vi "Host-Top-Level.vi"() -> ()   [LabVIEW 2017]
uses:
  State.ctl
  <vilib>/FPGAPlugInAG/PXIe-6592R/niLvFpga_Open_PXIe-6592R.vi
  <vilib>/rvi/interface/common/dynamic/niFpgaDynamicAddResources.vi
  <vilib>/Utility/error.llb/Error Cluster From Error Code.vi
  <vilib>/rvi/errors/niLvFpgaAdjustHostInterfaceError.vi
  <vilib>/FPGAPlugInAG/Dynamic/niLvFpga_Close_Dynamic.vi
  <vilib>/rvi/interface/nirviOpenFPGA/nirviOpenFPGA.xnode
  FPGA Bitfiles/04lwIpExercisor_FPGATarget_Fpga-Exercisor-T_vFkl61iGjK8.lvbitx
  PXIe-6592/Fpga-Exercisor-Top.vi
  <vilib>/rvi/interface/nirviMethod/nirviMethod.xnode
  <vilib>/rvi/interface/nirviReadWriteControl/nirviReadWriteControl.xnode
  <vilib>/rvi/interface/nirviCloseFPGA/nirviCloseFPGA.xnode
  <vilib>/rvi/errors/niLvFpgaMergeErrorWithErrorCode.vi
  <vilib>/FPGAPlugInAG/Dynamic/niLvFpga_ReadFifo_Dynamic.vi
  <vilib>/rvi/interface/Simulation/niFpgaSimulationCallBeginRW.vi
  <vilib>/FPGAPlugInAG/Dynamic/niLvFpga_WriteFifo_Dynamic.vi
  NiFpgaLv.dll
panel:
  in  "Read FIFO #2":bool
  in  "Read FIFO #1":bool
  in  "Interrupt #1":bool
  in  "Interrupt #0":bool
  out "AXI_STR_RXD_tready 2":bool
  out "tvalid 2":bool
  out "tdata 2":u32
  out "tlast 2":bool
  out "AXI_STR_RXD_tready_Count 2":u16
  out "tvalid_Count 2":u16
  out "tlast_Count 2":u16
  out "tdata_LastNonZero 2":u32
  out "Read Data 2":u32[](array[numeric]) format="%.0x"
  in  "DataToSend 2":u32[](array[numeric])=[240, 241, 242, 243, 244, 245] format="%.0x"
  in  "Send to FIFO #2":bool
  out "GPO2 Channel 2":u32
  in  "GPO2 Channel 1":u32
  in  "GPIO Write-Read #2":bool
  out "GPO1 Channel 1":u32 format="%.0x"
  out "error out":errorcluster
  out "GPO2 Channel 2":u32 format="%.0x"
  in  "Read all GPO":bool
  out "GPO1 Channel 2":u32
  in  "GPO1 Channel 1":u32
  in  "GPIO Write-Read #1":bool
  out "Read Data":u32[](array[numeric]) format="%.0x"
  in  "DataToSend":u32[](array[numeric])=[240, 241, 242, 243, 244, 245] format="%.0x"
  in  "Send to FIFO #1":bool
  in  "Stop":bool
  in  "error in":errorcluster
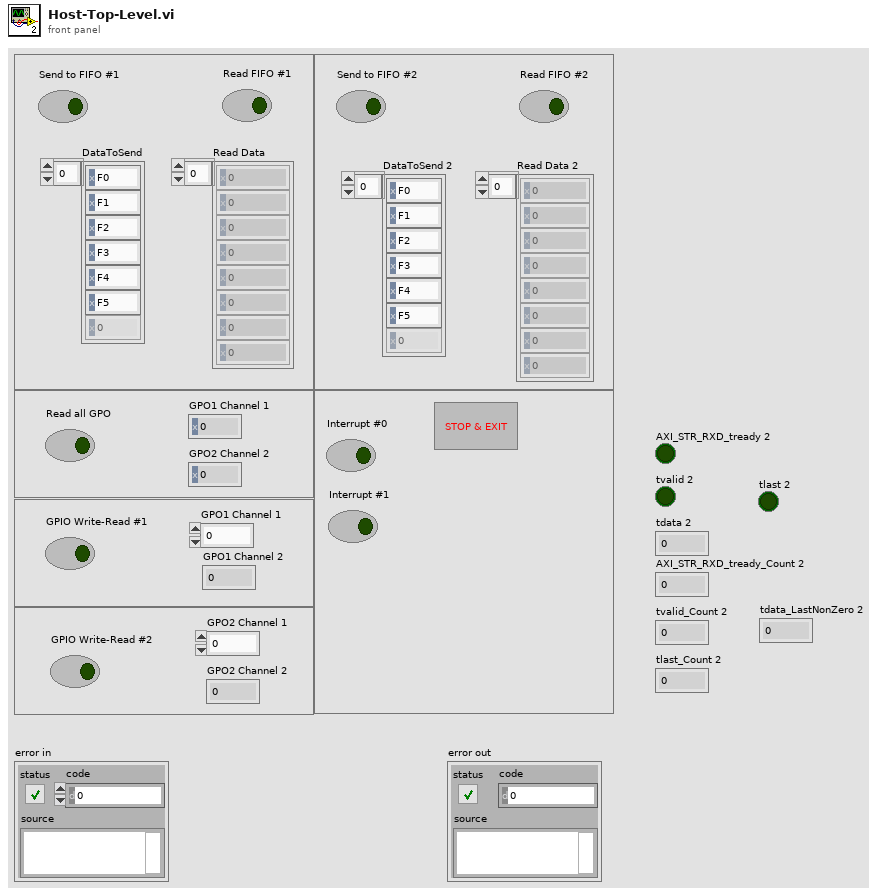
[diagram p1: front panel]
types:
  T1 = typedef "State.ctl" = enum16{"Initialize", "Idle", "Read #1", "Read #2", "Read Status", "Exit"}
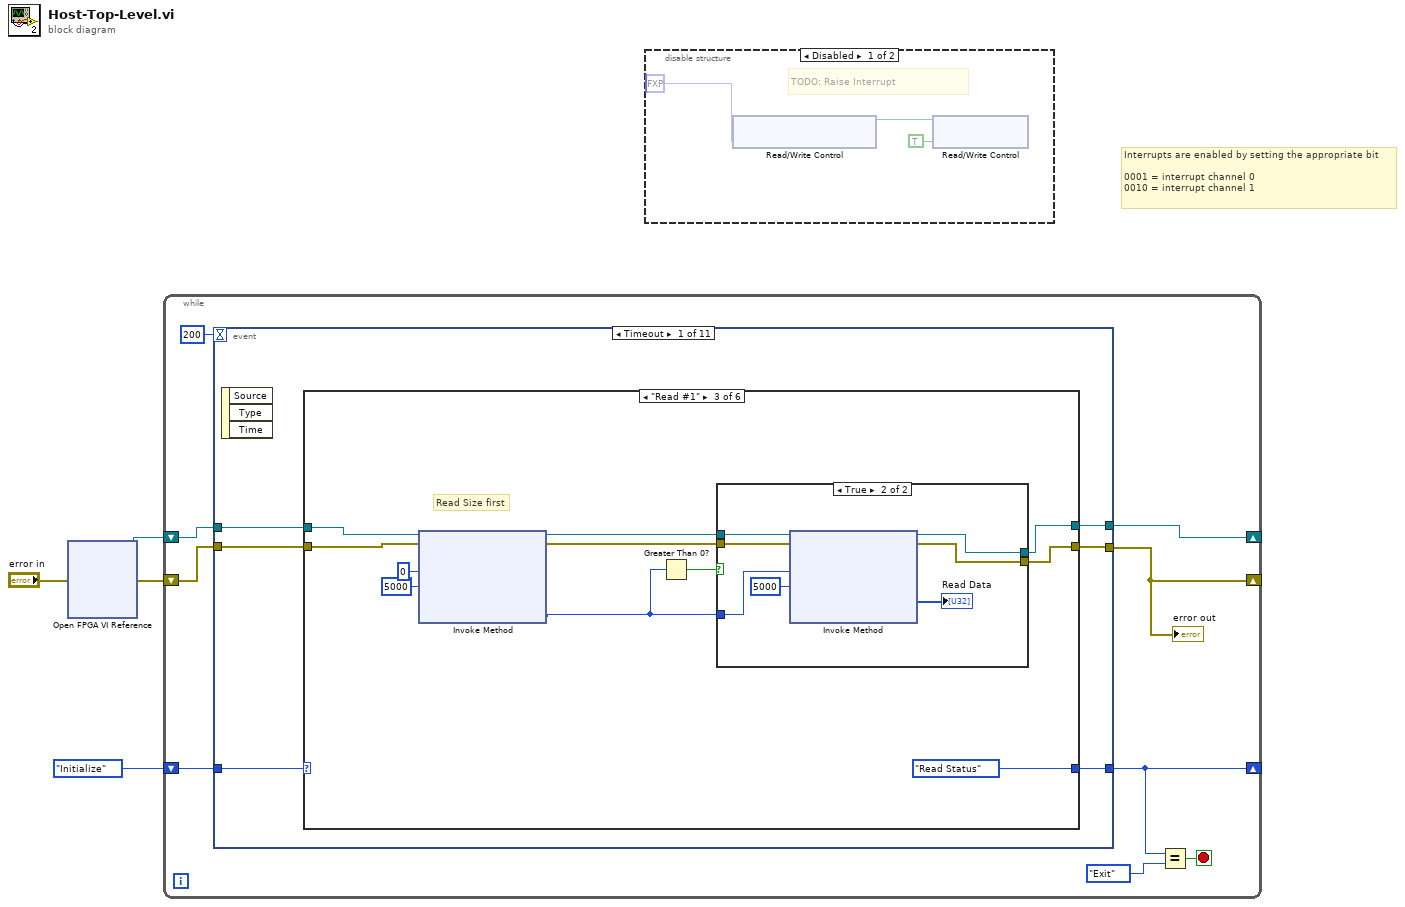
[diagram p0: block diagram]
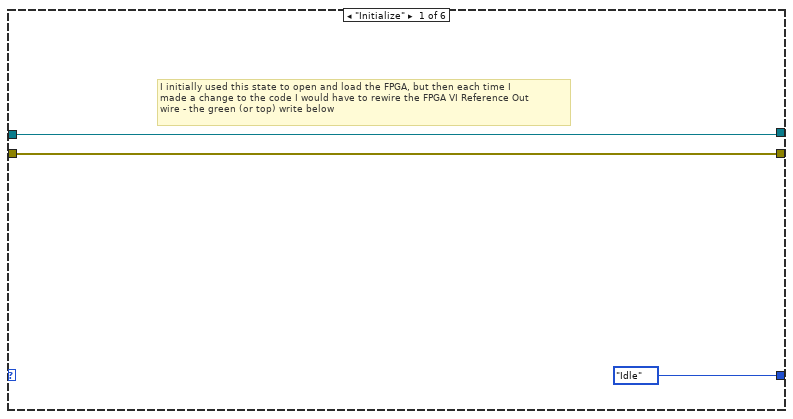
[diagram p3: hidden frame]
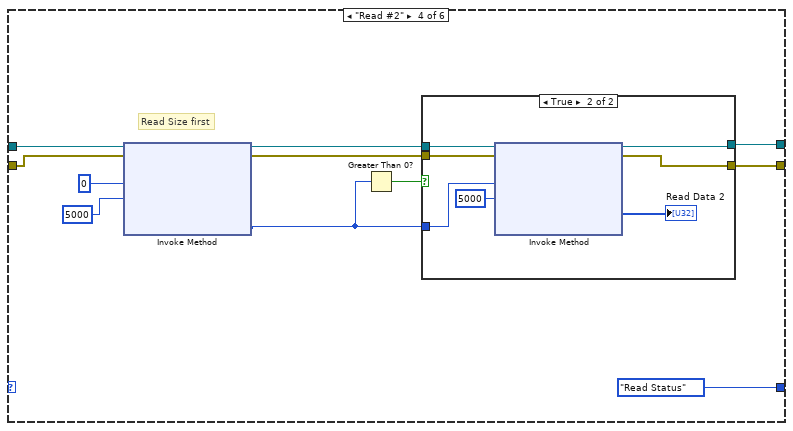
[diagram p6: hidden frame]
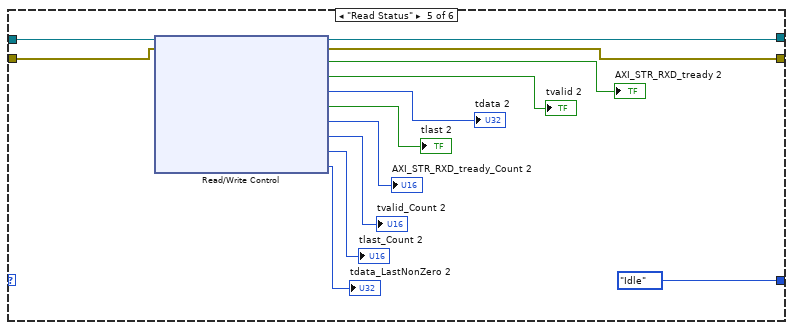
[diagram p8: hidden frame]
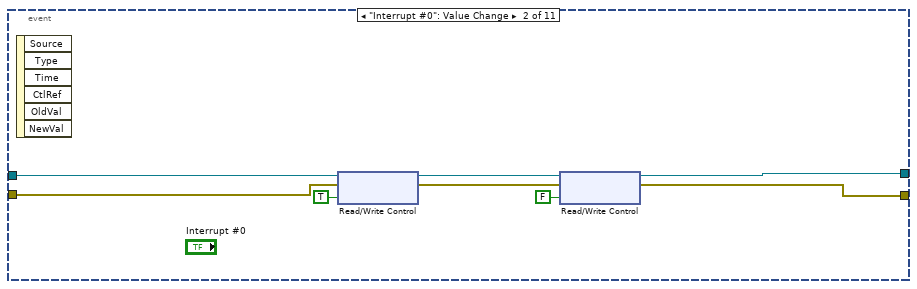
[diagram p10: hidden frame]
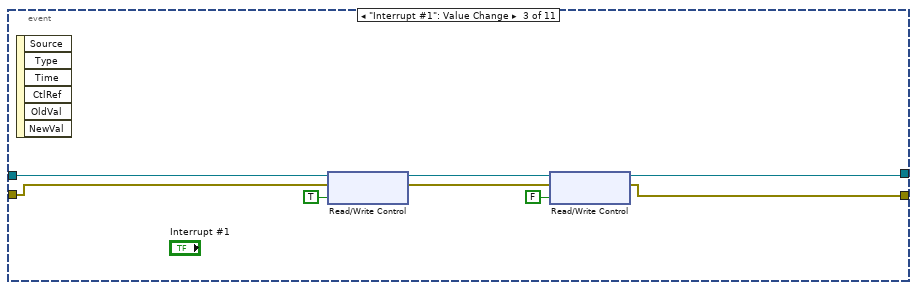
[diagram p11: hidden frame]
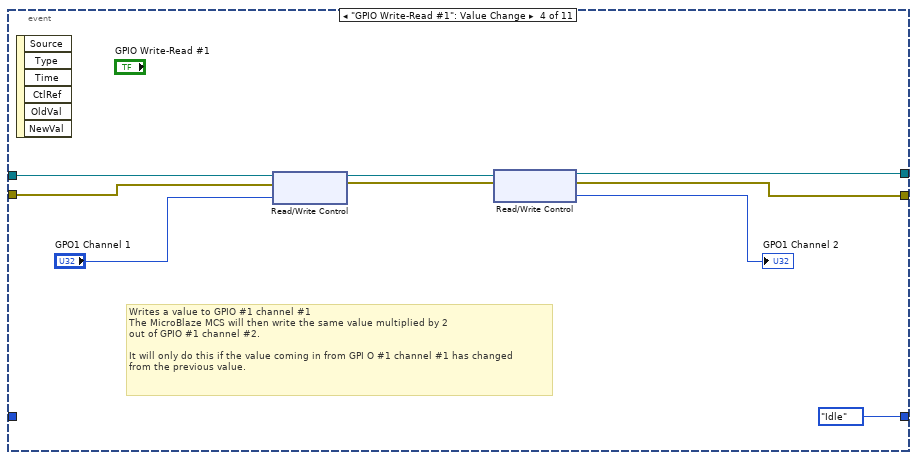
[diagram p12: hidden frame]
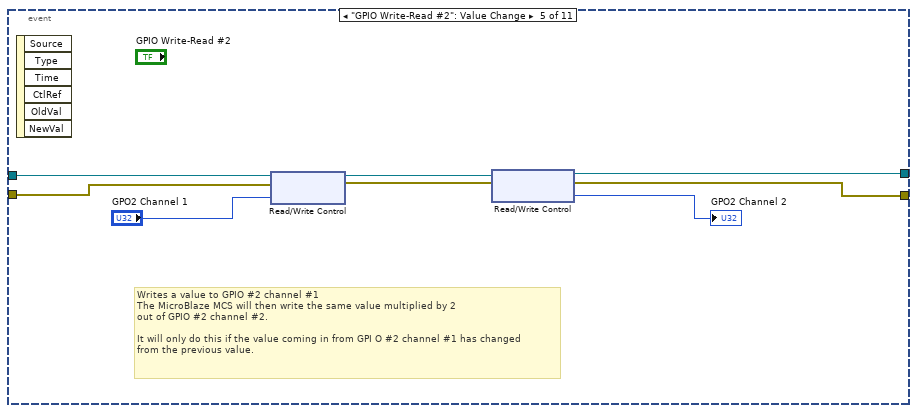
[diagram p13: hidden frame]
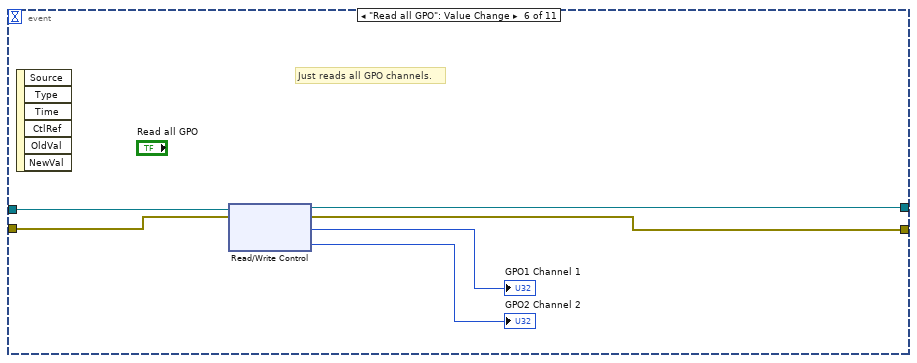
[diagram p14: hidden frame]
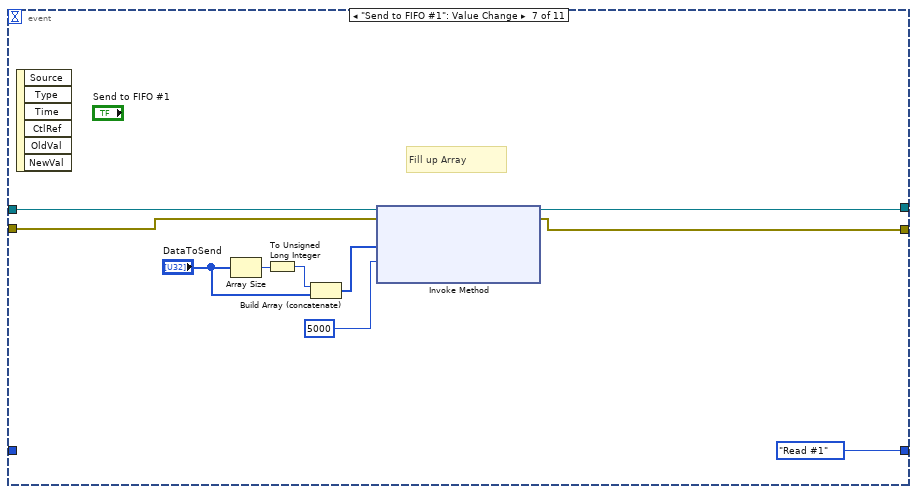
[diagram p15: hidden frame]
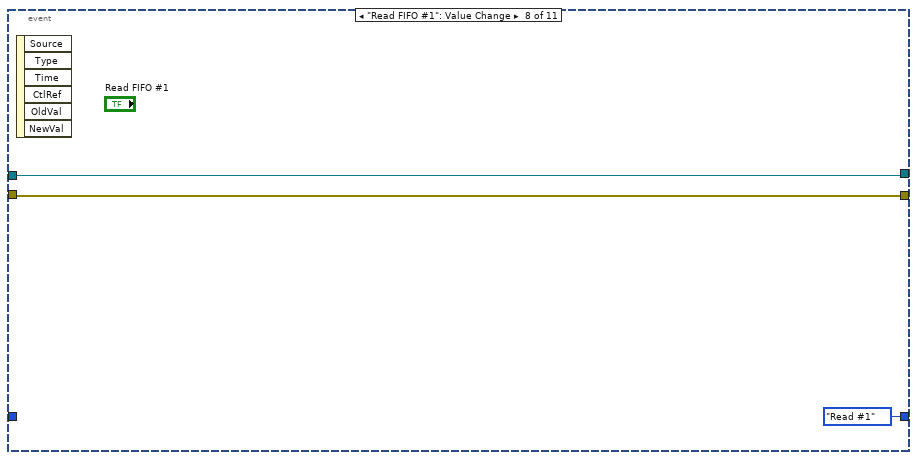
[diagram p16: hidden frame]
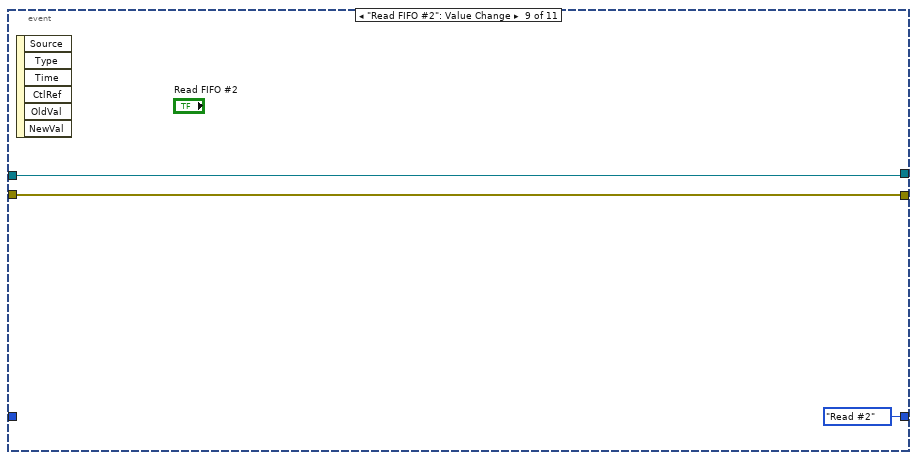
[diagram p17: hidden frame]
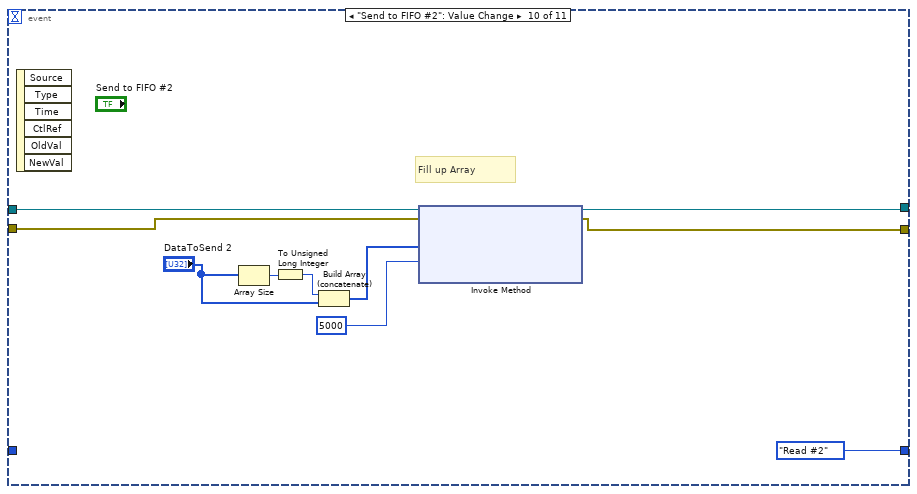
[diagram p18: hidden frame]
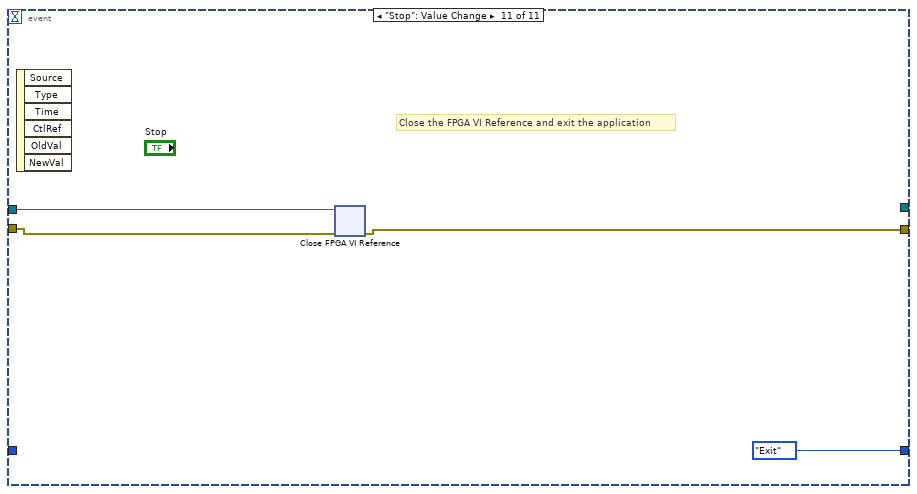
[diagram p19: hidden frame]
diagram:
  # "Interrupts are enabled by setting the appropriate bit\n\n0001 = interrupt channel 0\n0010 = interrupt channel 1"
  n1 = xnode "Open FPGA VI Reference"("error in"="error in") -> ("FPGA VI Reference Out"=w4:refnum<k20>, "error out"=w2:errorcluster)  [unwired: 1 in]
  n2 = while {
    shift-right: [w7] -> _
    shift-left: State."Initialize" ("Enum") -> [w13]
    shift-right: [w8] -> _
    shift-left: w2 -> [w9]
    shift-right: [w6] -> _
    shift-left: w4 -> [w5]
    stop <- w11 stop-if-true
    n3 = event shown="[0] Timeout" {
      selector: _ -> [_ _ _ _ _ _ _ _ _ _ _]
      dyn-events: _ -> [_ _ _ _ _ _ _ _ _ _ _]
      timeout: 200 -> [_ _ _ _ _ _ _ _ _ _ _]
      tunnel: [w17 _ _ State."Idle" ("Enum") _ _ State."Read #1" ("Enum") State."Read #1" ("Enum") State."Read #2" ("Enum") State."Read #2" ("Enum") State."Exit" ("Enum")] -> w7
      tunnel: w13 -> [w16 _ _ _ _ _ _ _ _ _ _]
      tunnel: w5 -> [w15 w89 w93 w105 w112 w120 w130 w132 w134 w146 w150]
      tunnel: w9 -> [w19 w83 w92 w104 w111 w119 w129 w131 w135 w145 w149]
      tunnel: [w18 w84 w91 w100 w110 w118 w122 w131 w135 w138 w148] -> w8
      tunnel: [w14 w85 w90 w98 w107 w117 w121 w132 w134 w139 _] -> w6
      event Timeout {
        n4 = event-data() -> ()  [unwired: 1 in, 3 out]
        n5 = case shown="\"Read #1\"" w16 {
          selector: w16 -> [_ w24 _ _ _ w80]
          tunnel: w19 -> [w21 w25 w36 w56 w68 w81]
          tunnel: [w21 w25 w31 w51 w67 w81] -> w18
          tunnel: w15 -> [w20 w23 w27 w47 w77 w79]
          tunnel: [State."Idle" ("Enum") w24 State."Read Status" ("Enum") State."Read Status" ("Enum") State."Idle" ("Enum") w80] -> w17
          tunnel: [w20 w23 w28 w48 w66 w79] -> w14
          frame "Initialize" {
            # "I initially used this state to open and load the FPGA, but then each time I \nmade a change to the code I would have to rewire the FPGA VI Reference Out \nwire - the green (or top) write below"
          }
          frame "Idle", Default {
          }
          frame "Read #1" {
            # "Read Size first"
            n6 = xnode "Invoke Method"("FPGA VI Reference In"=w27, "error in"=w36, "Number of Elements"=u32 0, "Timeout (ms)"=5000) -> ("FPGA VI Reference Out"=w32:refnum<k20>, "error out"=w33:errorcluster, "Elements Remaining"=w26:u32)  [unwired: 1 out]
            n7 = Greater Than 0?(x=w26) -> (x > 0?=w29:bool)
            n8 = case shown="True" w29 {
              tunnel: w33 -> [w38 w45]
              tunnel: w32 -> [w37 w44]
              tunnel: [w38 w42] -> w31
              tunnel: [w37 w41] -> w28
              tunnel: w26 -> [_ w39]
              frame False {
              }
              frame True {
                n9 = xnode "Invoke Method"("FPGA VI Reference In"=w44, "error in"=w45, "Number of Elements"=w39, "Timeout (ms)"=5000) -> ("FPGA VI Reference Out"=w41:refnum<k20>, "error out"=w42:errorcluster, "Data"=→"Read Data":u32[])  [unwired: 1 out]
              }
            }
          }
          frame "Read #2" {
            # "Read Size first"
            n10 = xnode "Invoke Method"("FPGA VI Reference In"=w47, "error in"=w56, "Number of Elements"=u32 0, "Timeout (ms)"=5000) -> ("FPGA VI Reference Out"=w52:refnum<k20>, "error out"=w53:errorcluster, "Elements Remaining"=w46:u32)  [unwired: 1 out]
            n11 = Greater Than 0?(x=w46) -> (x > 0?=w49:bool)
            n12 = case shown="True" w49 {
              tunnel: w53 -> [w58 w65]
              tunnel: w52 -> [w57 w64]
              tunnel: [w58 w62] -> w51
              tunnel: [w57 w61] -> w48
              tunnel: w46 -> [_ w60]
              frame False {
              }
              frame True {
                n13 = xnode "Invoke Method"("FPGA VI Reference In"=w64, "error in"=w65, "Number of Elements"=w60, "Timeout (ms)"=5000) -> ("FPGA VI Reference Out"=w61:refnum<k20>, "error out"=w62:errorcluster, "Data"=→"Read Data 2":u32[])  [unwired: 1 out]
              }
            }
          }
          frame "Read Status" {
            n14 = xnode "Read/Write Control"("FPGA VI Reference In"=w77, "error in"=w68) -> ("FPGA VI Reference Out"=w66:refnum<k20>, "error out"=w67:errorcluster, "AXI_STR_RXD_tready 2"=→"AXI_STR_RXD_tready 2":bool, "tvalid 2"=→"tvalid 2":bool, "tdata 2"=→"tdata 2":u32, "tlast 2"=→"tlast 2":bool, "AXI_STR_RXD_tready_Count 2"=→"AXI_STR_RXD_tready_Count 2":u16, "tvalid_Count 2"=→"tvalid_Count 2":u16, "tlast_Count 2"=→"tlast_Count 2":u16, "tdata_LastNonZero 2"=→"tdata_LastNonZero 2":u32)
          }
          frame "Exit" {
          }
        }
      }
      event "Interrupt #0": Value Change {
        n15 = event-data() -> ()  [unwired: 1 in, 6 out]
        n16 = xnode "Read/Write Control"("FPGA VI Reference In"=w89, "error in"=w83, "Interrupt #0"=TRUE) -> ("FPGA VI Reference Out"=w86:refnum<k20>, "error out"=w82:errorcluster)
        n17 = xnode "Read/Write Control"("FPGA VI Reference In"=w86, "error in"=w82, "Interrupt #0"=FALSE) -> ("FPGA VI Reference Out"=w85:refnum<k20>, "error out"=w84:errorcluster)
      }
      event "Interrupt #1": Value Change {
        n18 = event-data() -> ()  [unwired: 1 in, 6 out]
        n19 = xnode "Read/Write Control"("FPGA VI Reference In"=w93, "error in"=w92, "Interrupt #1"=TRUE ("Interrupt #0")) -> ("FPGA VI Reference Out"=w95:refnum<k20>, "error out"=w94:errorcluster)
        n20 = xnode "Read/Write Control"("FPGA VI Reference In"=w95, "error in"=w94, "Interrupt #1"=FALSE ("Interrupt #0")) -> ("FPGA VI Reference Out"=w90:refnum<k20>, "error out"=w91:errorcluster)
      }
      event "GPIO Write-Read #1": Value Change {
        # "Writes a value to GPIO #1 channel #1\nThe MicroBlaze MCS will then write the same value multiplied by 2\nout of GPIO #1 channel #2.\n\nIt will only do this if the value coming in from GPI O #1 channel #1 has changed\nfrom the previous value."
        n21 = event-data() -> ()  [unwired: 1 in, 6 out]
        n22 = xnode "Read/Write Control"("FPGA VI Reference In"=w105, "error in"=w104, "GPIO #1 in"="GPO1 Channel 1") -> ("FPGA VI Reference Out"=w99:refnum<k20>, "error out"=w102:errorcluster)
        n23 = xnode "Read/Write Control"("FPGA VI Reference In"=w99, "error in"=w102) -> ("FPGA VI Reference Out"=w98:refnum<k20>, "error out"=w100:errorcluster, "GPIO #1 out"=→"GPO1 Channel 2":u32)
      }
      event "GPIO Write-Read #2": Value Change {
        # "Writes a value to GPIO #2 channel #1\nThe MicroBlaze MCS will then write the same value multiplied by 2\nout of GPIO #2 channel #2.\n\nIt will only do this if the value coming in from GPI O #2 channel #1 has changed\nfrom the previous value."
        n24 = event-data() -> ()  [unwired: 1 in, 6 out]
        n25 = xnode "Read/Write Control"("FPGA VI Reference In"=w112, "error in"=w111, "GPIO #2 in"="GPO2 Channel 1") -> ("FPGA VI Reference Out"=w113:refnum<k20>, "error out"=w114:errorcluster)
        n26 = xnode "Read/Write Control"("FPGA VI Reference In"=w113, "error in"=w114) -> ("FPGA VI Reference Out"=w107:refnum<k20>, "error out"=w110:errorcluster, "GPIO #2 out"=→"GPO2 Channel 2":u32)
      }
      event "Read all GPO": Value Change {
        # "Just reads all GPO channels."
        n27 = event-data() -> ()  [unwired: 1 in, 6 out]
        n28 = xnode "Read/Write Control"("FPGA VI Reference In"=w120, "error in"=w119) -> ("FPGA VI Reference Out"=w117:refnum<k20>, "error out"=w118:errorcluster, "GPIO #1 out"=→"GPO1 Channel 1":u32, "GPIO #2 out"=→"GPO2 Channel 2":u32)
      }
      event "Send to FIFO #1": Value Change {
        # "Fill up Array"
        n29 = event-data() -> ()  [unwired: 1 in, 6 out]
        n30 = Array Size(array="DataToSend") -> (size(s)=w128:i32)
        n31 = To Unsigned Long Integer(number=w128) -> (unsigned 32bit integer=w125:u32)
        n32 = Build Array (concatenate)(w125, "DataToSend") -> (w126:u32[])
        n33 = xnode "Invoke Method"("FPGA VI Reference In"=w130, "error in"=w129, "Data"=w126, "Timeout (ms)"=5000) -> ("FPGA VI Reference Out"=w121:refnum<k20>, "error out"=w122:errorcluster)  [unwired: 1 out]
      }
      event "Read FIFO #1": Value Change {
        n34 = event-data() -> ()  [unwired: 1 in, 6 out]
      }
      event "Read FIFO #2": Value Change {
        n35 = event-data() -> ()  [unwired: 1 in, 6 out]
      }
      event "Send to FIFO #2": Value Change {
        # "Fill up Array"
        n36 = event-data() -> ()  [unwired: 1 in, 6 out]
        n37 = Array Size(array="DataToSend 2") -> (size(s)=w144:i32)
        n38 = To Unsigned Long Integer(number=w144) -> (unsigned 32bit integer=w142:u32)
        n39 = Build Array (concatenate)(w142, "DataToSend 2") -> (w143:u32[])
        n40 = xnode "Invoke Method"("FPGA VI Reference In"=w146, "error in"=w145, "Data"=w143, "Timeout (ms)"=5000) -> ("FPGA VI Reference Out"=w139:refnum<k20>, "error out"=w138:errorcluster)  [unwired: 1 out]
      }
      event "Stop": Value Change {
        # "Close the FPGA VI Reference and exit the application"
        n41 = event-data() -> ()  [unwired: 1 in, 6 out]
        n42 = xnode "Close FPGA VI Reference"("FPGA VI Reference In"=w150, "error in"=w149) -> ("error out"=w148:errorcluster)
      }
    }
    "error out" <- w8
    n43 = Equal?(x=w7, y=State."Exit") -> (x = y?=w11:bool)
  }
  n44 = disable-structure shown="Disabled" {
    frame Disabled {
      # "TODO: Raise Interrupt"
      n45 = xnode "Read/Write Control"("d_mcs_i\\INTC_Interrupt"=fxp<+,4,4> 1.0 ("Interrupt Number")) -> ("FPGA VI Reference In"=w154:refnum<k20>, "FPGA VI Reference Out"=w152:refnum<k20>)  [unwired: 1 in, 1 out]
      n46 = xnode "Read/Write Control"("FPGA VI Reference In"=w152, "Write Interrupt"=TRUE) -> ()  [unwired: 1 in, 2 out]
    }
    frame Enabled {
    }
  }
